vi "Concatenate result strings.vi"(9 "Description":string, 10 "Status":T1=enum."Passed", 11 "Input String":string) -> (3 "Output String":string)   [LabVIEW 2020, in "LUnit Test Case.lvclass"]
uses:
  LUnit Test Case.lvclass
  LUnit Test Case.lvclass/LUnit Test Case.ctl
  Result/Status.ctl
  Result/Result.lvlib
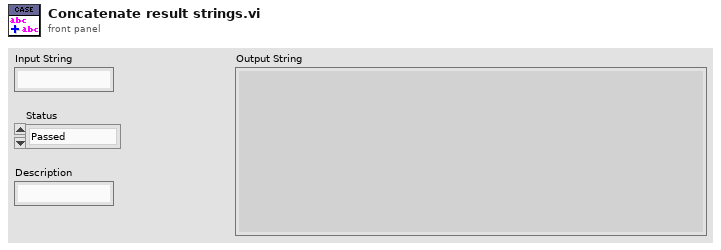
[diagram p1: front panel]
types:
  T1 = typedef "Result.lvlib/Status.ctl" = enum16{"", "Passed", "Failed", "Error", "Skipped", "Setup Error", "Broken", "Teardown Error"}
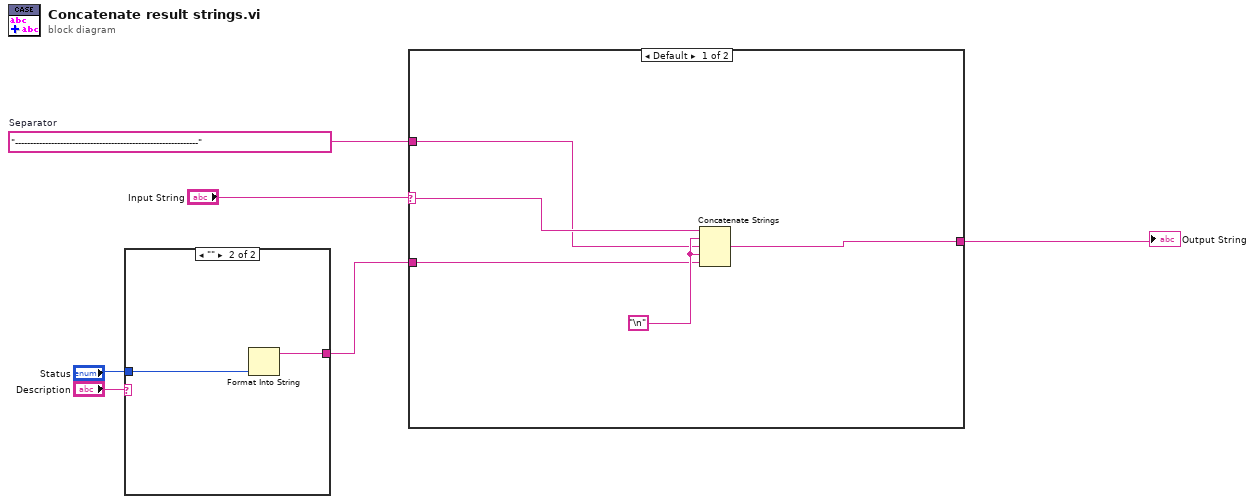
[diagram p0: block diagram]
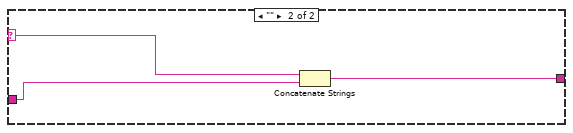
[diagram p2: hidden frame]
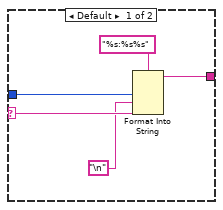
[diagram p3: hidden frame]
diagram:
  w6 = "-------------------------------------------------------------"  # Separator
  n1 = case shown="\"\"" "Description" {
    selector: "Description" -> [w10 _]
    tunnel: "Status" -> [w11 w13]
    tunnel: [w9 w12] -> w2
    frame Default {
      n2 = Format Into String(format string="%s:%s%s", w11, "\n", w10) -> (resulting string=w9:string)  [unwired: 2 in, 1 out]
    }
    frame "" {
      n3 = Format Into String(w13) -> (resulting string=w12:string)  [unwired: 3 in, 1 out]
    }
  }
  n4 = case shown="Default" "Input String" {
    selector: "Input String" -> [w17 w19]
    tunnel: w2 -> [w15 w21]
    tunnel: w6 -> [w14 _]
    tunnel: [w18 w20] -> w1
    frame Default {
      w16 = "\n"
      n5 = Concatenate Strings(w17, w16, w14, w16, w15) -> (w18:string)
    }
    frame "" {
      n6 = Concatenate Strings(w19, w21) -> (w20:string)
    }
  }
  "Output String" <- w1
